vi "ENA_status.vi"(8 "error in (no error)":errorcluster caption="错误输入（无错误）", 11 "StepMotor 输入":refnum<class "StepMotor.lvclass">) -> (0 "error out":errorcluster caption="错误输出", 2 "ENA status":bool, 3 "StepMotor 输出":refnum<class "StepMotor.lvclass">)   [LabVIEW 2016, in "MotionControl.lvlib" / "StepMotor.lvclass"]
uses:
  <userlib>/MotionControl/StepMotor/StepMotor.lvclass
  <userlib>/MotionControl/StepMotor/StepMotor.lvclass/StepMotor.ctl
  <userlib>/UISimCanFunc_wrapper/UISimCanFunc_wrapper.lvlib
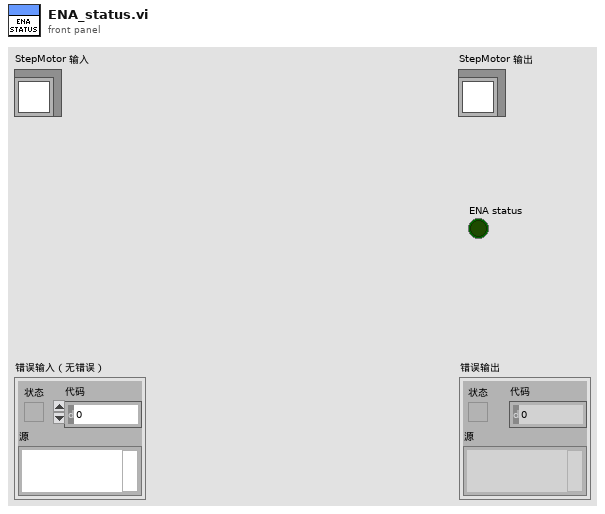
[diagram p1: front panel]
types:
  T1 = typedef "UISimCanFunc_wrapper.lvlib/BASIC_FBK_OBJ.ctl" = cluster{"uiReserv":u32, "bENA":bool, "bDIR":bool, "bACR":bool, "uiMCS":u32, "uiCUR":u32, "iSPD":i32, "iSTP":i32}
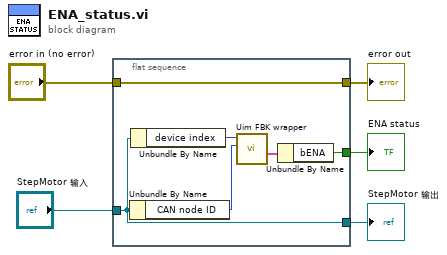
[diagram p0: block diagram]
diagram:
  n1 = flat-sequence {
    tunnel: "StepMotor 输入" -> [w7]
    tunnel: [w8] -> w4
    tunnel: [w7] -> w3
    tunnel: "error in (no error)" -> [w6]
    tunnel: [w6] -> w1
    frame #0 {
      n2 = Unbundle By Name(w7) -> ("CAN node ID"=w10:u32)
      n3 = Unbundle By Name(w7) -> ("device index"=w11:u32)
      n4 = call <userlib>:"Uim FBK wrapper.vi"("dwCanNodeId"=w10, "dwDevIndex"=w11) -> ("BASIC_FBK_OBJ"=w9:T1)  [unwired: 7 in, 2 out]
      n5 = Unbundle By Name(w9) -> ("bENA"=w8:bool)
    }
  }
  "error out" <- w1
  "StepMotor 输出" <- w3
  "ENA status" <- w4
